vi "Set message.vi"(10 "WampMessage MsgPack":refnum<class "WampMessage MsgPack.lvclass">, 11 "ResultHandler MsgPack in":refnum<class "ResultHandler MsgPack.lvclass">) -> (3 "ResultHandler MsgPack out":refnum<class "ResultHandler MsgPack.lvclass">)   [LabVIEW 2020, in "wamplv.lvlib" / "ResultHandler MsgPack.lvclass"]
uses:
  ResultHandler MsgPack.lvclass
  ResultHandler MsgPack.lvclass/ResultHandler MsgPack.ctl
  SerialisedMessages/MsgPackMessage/WampMessage MsgPack.lvclass
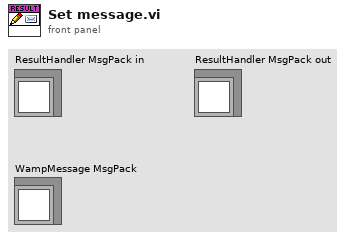
[diagram p1: front panel]
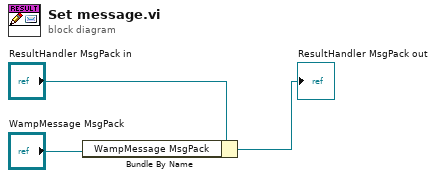
[diagram p0: block diagram]
diagram:
  n1 = Bundle By Name(cluster="ResultHandler MsgPack in", "WampMessage MsgPack"="WampMessage MsgPack") -> (→"ResultHandler MsgPack out":refnum<class "ResultHandler MsgPack.lvclass">)
